vi "Get port Status.vi"(8 "error in (no error)":errorcluster, 10 "Puerto":dbl, 11 "Cypress in":refnum<class "Cypress.lvclass">) -> (0 "error out":errorcluster, 3 "Cypress out":refnum<class "Cypress.lvclass">)   [LabVIEW 2020, in "Cypress.lvclass"]
uses:
  Cypress.lvclass
  f508de2a-1931-4b72-addc-a30d1f9d24f8.vi
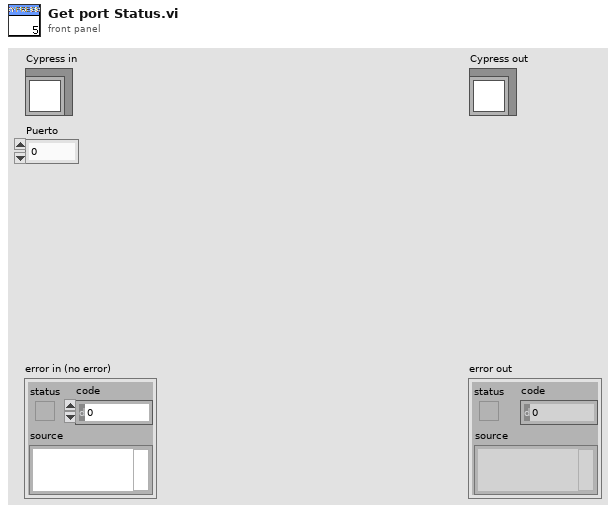
[diagram p1: front panel]
types:
  T1 = typedef "Serial Device.lvclass/serial device brand.ctl" = string
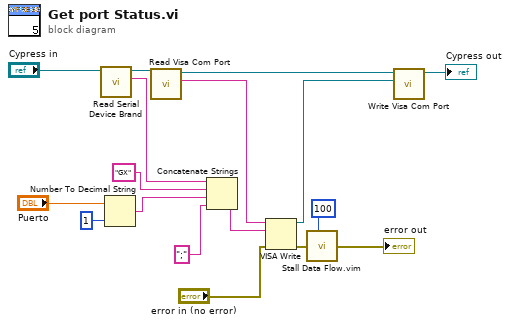
[diagram p0: block diagram]
diagram:
  n1 = call-dynamic "Read Serial Device Brand.vi"("Serial Device in"="Cypress in") -> ("Serial Device Brand"=w11:T1, "Serial Device out"=w14:refnum<class "Cypress.lvclass">)  [unwired: 8 in, 1 out]
  n2 = Number To Decimal String(number="Puerto", width (-)=i16 1) -> (decimal integer string=w9:string)
  n3 = call-dynamic "Read Visa Com Port.vi"("Serial Device in"=w14) -> ("Visa Com Port"=w5:string, "Serial Device out"=w13:refnum<class "Cypress.lvclass">)  [unwired: 8 in, 1 out]
  n4 = Concatenate Strings(w11, "GX" ("string"), w9, ";" ("string")) -> (w4:string)
  n5 = VISA Write(VISA resource name=w5, write buffer=w4, error in (no error)="error in (no error)") -> (VISA resource name out=w3:refnum<visa-resource-name>, error out=w17:errorcluster)  [unwired: 1 out]
  n6 = call "Stall Data Flow.vim"("value in"=w17, "milliseconds to wait"=u32 100) -> ("value out"=→"error out":errorcluster)  [unwired: 1 out]
  n7 = call-dynamic "Write Visa Com Port.vi"("Visa Com Port"=w3, "Serial Device in"=w13) -> ("Serial Device out"=→"Cypress out":refnum<class "Cypress.lvclass">)  [unwired: 8 in, 1 out]
